vi "Run Executable.vi"(0 "Folder":string, 5 ".EXE name":string, 7 "args":string[](array[string]), 9 "Wait (F)":bool, 11 "error in (no error)":errorcluster) -> (15 "error out":errorcluster)   [LabVIEW 2020]
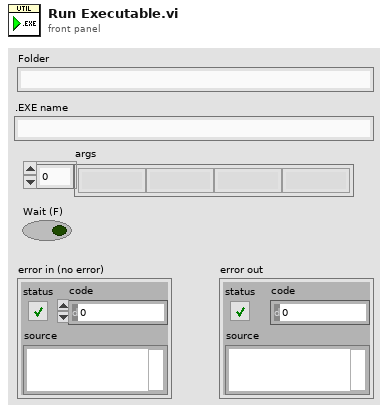
[diagram p1: front panel]
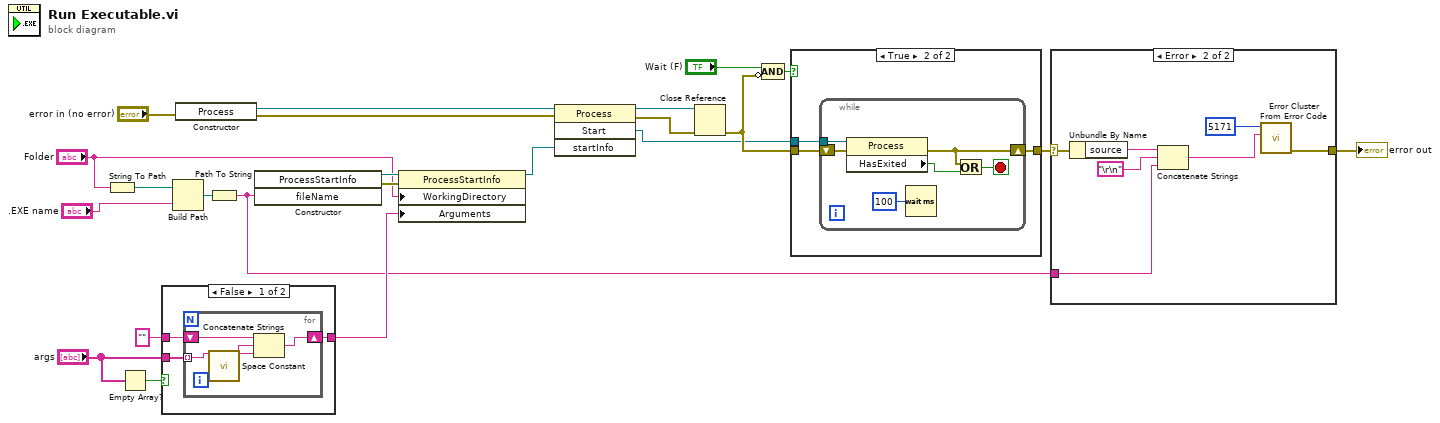
[diagram p0: block diagram]
diagram:
  n1 = String To Path(string="Folder") -> (path=w20:path)
  n2 = Empty Array?(array="args") -> (empty?=w16:bool)
  n3 = case shown="False" w16 {
    tunnel: "args" -> [w26 _]
    tunnel: "" -> [w25 w31]
    tunnel: [w24 w31] -> w4
    frame False {
      n4 = for {
        tunnel: w26 -> [w28] mode=indexing
        shift-right: [w29] -> w24
        shift-left: w25 -> [w30]
        n5 = call <vilib>:"Space Constant.vi"() -> ("String"=w27:string)
        n6 = Concatenate Strings(w30, w27, w28) -> (w29:string)
      }
    }
    frame True {
    }
  }
  n7 = Build Path(base path=w20, name or relative path=".EXE name") -> (appended path=w19:path)
  n8 = constructor class="Process"(error in="error in (no error)") -> (reference out=w23:refnum<k24>, error out=w22:errorcluster)  [unwired: 2 in, 1 out]
  n9 = Path To String(path=w19) -> (string=w2:string)
  n10 = constructor class="ProcessStartInfo"("fileName"=w2) -> (reference out=w7:refnum<k24>, error out=w8:errorcluster)  [unwired: 3 in, 2 out]
  n11 = property class="ProcessStartInfo"(reference=w7, error in=w8, "WorkingDirectory"="Folder", "Arguments"=w4) -> (reference out=w6:refnum<k24>)  [unwired: 1 out]
  n12 = invoke class="Process" method="Start"(reference=w23, error in=w22, "startInfo"=w6) -> (reference out=w11:refnum<k24>, error out=w12:errorcluster, "Start"=w9:refnum<k24>)  [unwired: 1 in, 1 out]
  n13 = Close Reference(reference=w11, error in (no error)=w12) -> (error out=w10:errorcluster)
  n14 = Compound Arithmetic op=AND("Wait (F)", invert w10) -> (w17:bool)
  n15 = case shown="True" w17 {
    tunnel: w10 -> [w32 w35]
    tunnel: [w32 w33] -> w3
    tunnel: w9 -> [_ w34]
    frame False {
    }
    frame True {
      n16 = while {
        tunnel: w34 -> [w41]
        shift-right: [w37] -> w33
        shift-left: w35 -> [w40]
        stop <- w38 stop-if-true
        n17 = property class="Process"(reference=w41, error in=w40) -> (error out=w37:errorcluster, "HasExited"=w39:bool)  [unwired: 1 out]
        n18 = Wait (ms)(milliseconds to wait=u32 100) -> ()  [unwired: 1 out]
        n19 = Or(x=w37, y=w39) -> (x .or. y?=w38:bool)
      }
    }
  }
  n20 = case shown="Error" w3 {
    selector: w3 -> [w42 w48]
    tunnel: w2 -> [_ w45]
    tunnel: [w42 w43] -> w1
    frame No Error {
    }
    frame Error {
      n21 = Unbundle By Name(w48) -> ("source"=w47:string)
      n22 = Concatenate Strings(w47, "\r\n", w45) -> (w44:string)
      n23 = call <vilib>:"Error Cluster From Error Code.vi"("error message (\"\")"=w44, "error code (0)"=5171) -> ("error out"=w43:errorcluster)  [unwired: 7 in]
    }
  }
  "error out" <- w1
